vi "Logger.CreateDirFromDate.vi"(8 "error in (no error)":errorcluster, 11 "base path":path) -> (0 "error out":errorcluster, 3 "Saving Dir":path)   [LabVIEW 2017]
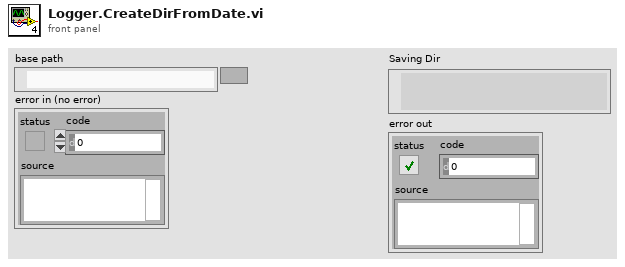
[diagram p1: front panel]
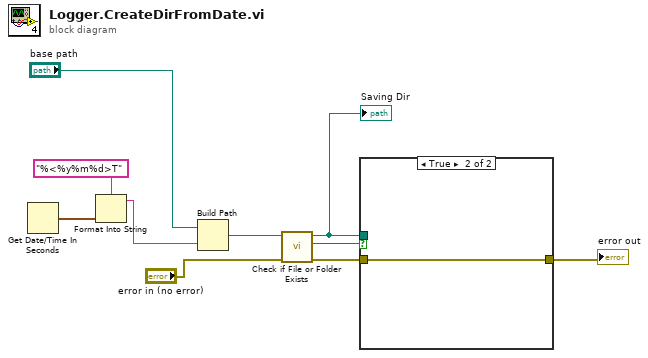
[diagram p0: block diagram]
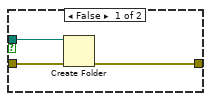
[diagram p2: hidden frame]
diagram:
  n1 = Get Date/Time In Seconds() -> (seconds since 1Jan1904=w10:timestamp)
  n2 = Format Into String(format string="%<%y%m%d>T", w10) -> (resulting string=w7:string)  [unwired: 2 in, 1 out]
  n3 = Build Path(base path="base path", name or relative path=w7) -> (appended path=w6:path)
  n4 = call <vilib>:"Check if File or Folder Exists.vi"("error in (no error)"="error in (no error)", "path"=w6) -> ("error out"=w3:errorcluster, "file or folder exists?"=w5:bool, "dup path"=w4:path)  [unwired: 7 in]
  "Saving Dir" <- w4
  n5 = case shown="True" w5 {
    tunnel: w4 -> [w13 _]
    tunnel: w3 -> [w12 w14]
    tunnel: [w11 w14] -> w1
    frame False {
      n6 = Create Folder(path (use dialog)=w13, error in=w12) -> (error out=w11:errorcluster)  [unwired: 1 in, 2 out]
    }
    frame True {
    }
  }
  "error out" <- w1
